vi "Set_Error.vi"(0 "CustomErrors":T1, 1 "SetError(True)":bool=TRUE, 2 "Description":string, 5 "error in (no error)":errorcluster) -> (19 "error out":errorcluster)   [LabVIEW 2019, in "LcWebView.lvclass"]
uses:
  LcWebView.lvclass
  ctrls/ErrorCode.ctl
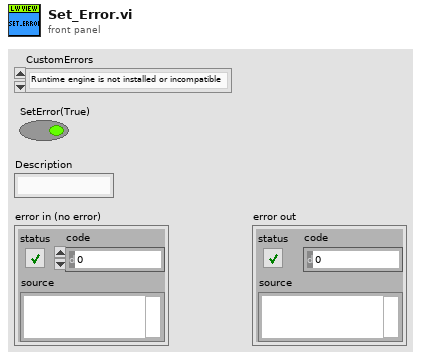
[diagram p1: front panel]
types:
  T1 = typedef "LcWebView.lvclass/ErrorCode.ctl" = enum16{"Runtime engine is not installed or incompatible", "User Data Folder cannot be set", "Others"}
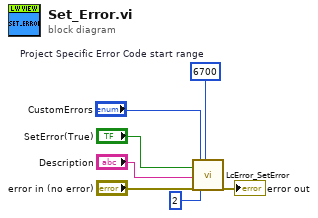
[diagram p0: block diagram]
diagram:
  w5 = 6700  # Project Specific Error Code start range
  n1 = call "LcError_SetError.vi"("status"="SetError(True)", "source"="Description", "error in (no error)"="error in (no error)", "UserDefinedCodes(+5000)"="CustomErrors", "Error SubVI Level(1)"=2, "StartErrorCode(5000)"=w5) -> ("error out"=→"error out":errorcluster)  [unwired: 13 in]
